vi "Get SQL formatted value.vi"(8 "error in (no error)":errorcluster, 11 "Column in":refnum<class "Text Field.lvclass">) -> (0 "error out":errorcluster, 2 "Formatted Value":string, 3 "Column out":refnum<class "Text Field.lvclass">)   [LabVIEW 2020]
uses:
  Basic Fields/Basic Field Class/Ctrl Refnum Column.lvclass
  Text Field.lvclass
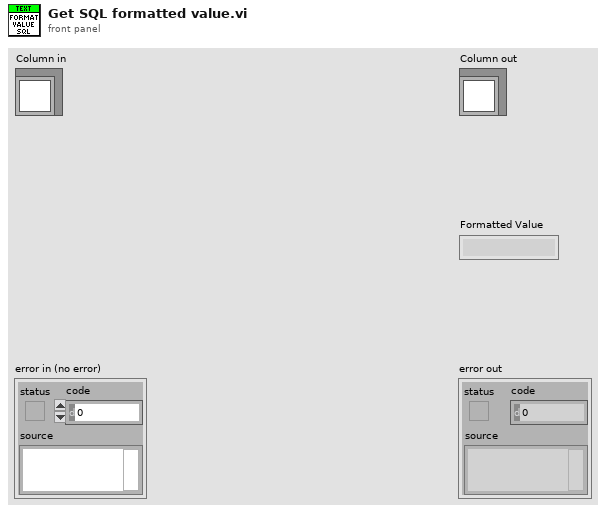
[diagram p1: front panel]
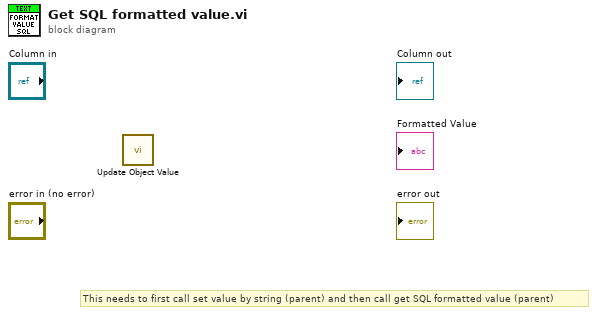
[diagram p0: block diagram]
diagram:
  # "This needs to first call set value by string (parent) and then call get SQL formatted value (parent)"
  n1 = call-dynamic "Update Object Value.vi"() -> ()  [unwired: 10 in, 2 out]
